vi "VI Server_Set Control Signaling Value from String Format.vi"(4 "milliseconds to wait (10 ms)":u32=10, 6 "New Signaling Value (String)":string, 7 "Label":string, 8 "error in (no error)":errorcluster, 11 "VI Server Cluster":T1={"Labels"=["Label", "Size", "Font", "Heght", "Width", "Ledding Denominator", "Ledding Nominator", "Label Number", "Microstep Resolution", "X", "Y", "Z", "Italic?", "Underlined?"], "Refs"=[], "VI Ref"=refnum}) -> (0 "error out":errorcluster, 3 "VI Server Cluster.DUP":T1={"Labels"=["Label", "Size", "Font", "Heght", "Width", "Ledding Denominator", "Ledding Nominator", "Label Number", "Microstep Resolution", "X", "Y", "Z", "Italic?", "Underlined?"], "Refs"=[], "VI Ref"=refnum})   [LabVIEW 2020, in "VI Server Toolkit LV2013.lvlib"]
doc: "<B>Set Control Values From String Formats.vi</B> and converts string values of the selected GUI objects onto original data type.\nInserts value change event into Windows Events Queue."
uses:
  VI Server Toolkit LV2013.lvlib
  VI Server_TypeDefs/VI Server_RefsCluster.ctl
panel:
  in  "Path":refnum<vi>
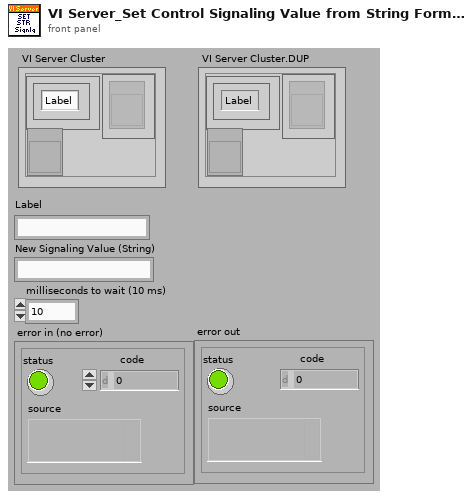
[diagram p1: front panel]
types:
  T1 = typedef "VI Server_RefsCluster.ctl" = cluster{"Labels":string[], "Refs":refnum<vi>[], "VI Ref":refnum<vi>}
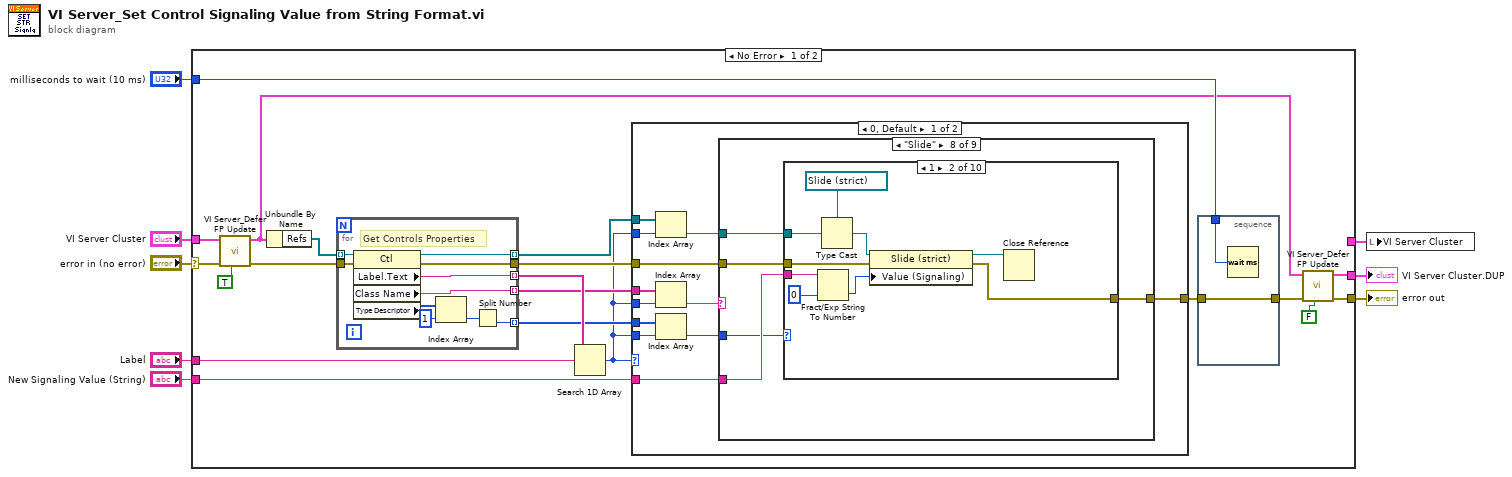
[diagram p0: block diagram]
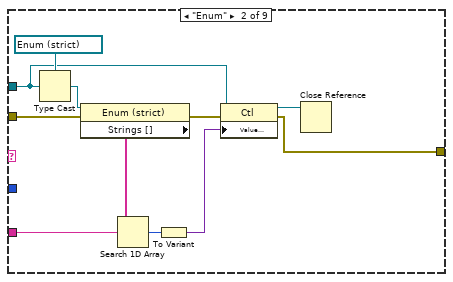
[diagram p3: hidden frame]
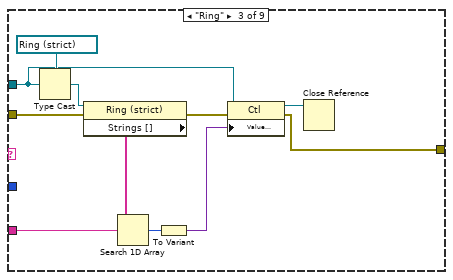
[diagram p4: hidden frame]
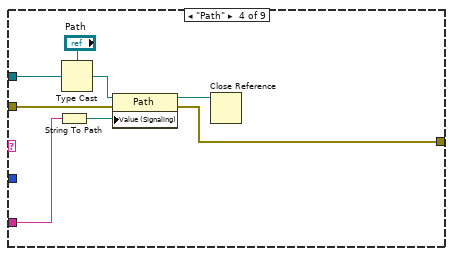
[diagram p5: hidden frame]
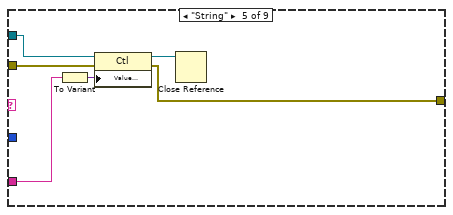
[diagram p6: hidden frame]
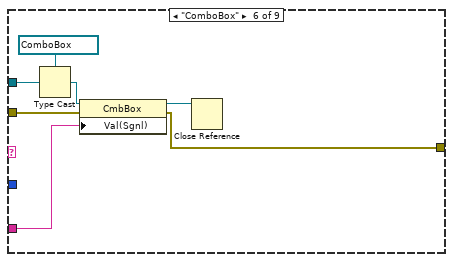
[diagram p7: hidden frame]
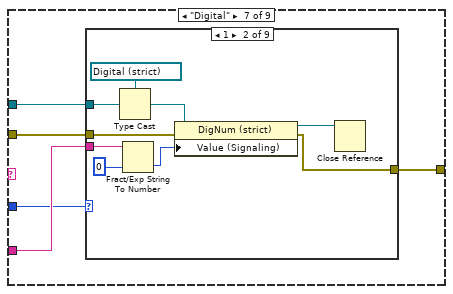
[diagram p8: hidden frame]
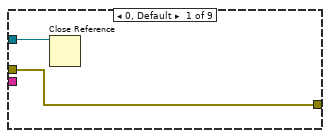
[diagram p9: hidden frame]
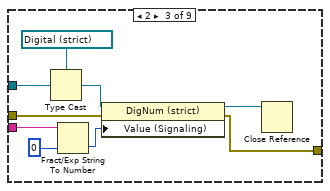
[diagram p10: hidden frame]
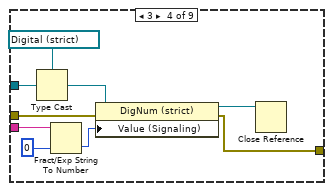
[diagram p11: hidden frame]
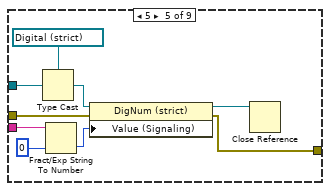
[diagram p12: hidden frame]
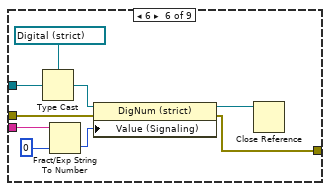
[diagram p13: hidden frame]
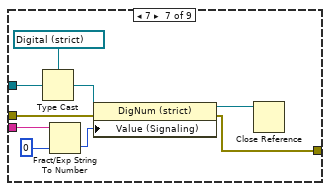
[diagram p14: hidden frame]
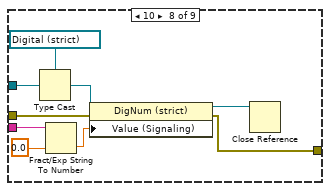
[diagram p15: hidden frame]
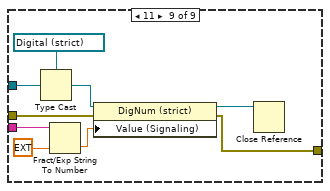
[diagram p16: hidden frame]
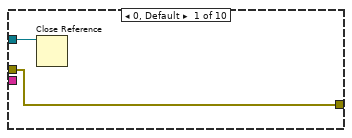
[diagram p17: hidden frame]
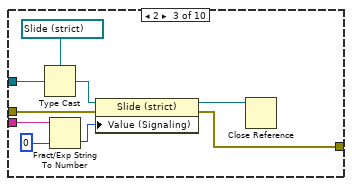
[diagram p18: hidden frame]
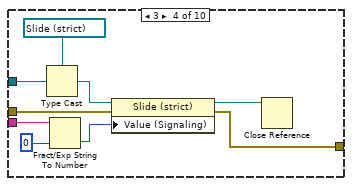
[diagram p19: hidden frame]
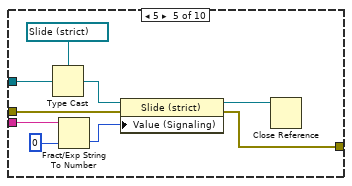
[diagram p20: hidden frame]
diagram:
  n1 = case shown="No Error" "error in (no error)" {
    selector: "error in (no error)" -> [w21 w275]
    tunnel: "New Signaling Value (String)" -> [w23 _]
    tunnel: [w17 w275] -> w8
    tunnel: "VI Server Cluster" -> [w19 _]
    tunnel: "milliseconds to wait (10 ms)" -> [w14 _]
    tunnel: "Label" -> [w13 _]
    tunnel: [w9 _] -> w2
    tunnel: [_ w274] -> w1
    frame No Error {
      n2 = call "VI Server_Defer FP Update.vi"("Defer Panel Updates? (F)"=TRUE ("Defer Panel Updates (F)"), "error in"=w21, "VI Server Cluster"=w19) -> ("error out"=w20:errorcluster, "VI Server Cluster.DUP"=w10:T1)  [unwired: 7 out]
      n3 = Unbundle By Name(w10) -> ("Refs"=w22:refnum<vi>[])
      n4 = for {
        tunnel: w22 -> [w273] mode=indexing
        tunnel: w20 -> [w272]
        tunnel: [w271] -> w28 mode=indexing
        tunnel: [w270] -> w26 mode=indexing
        tunnel: [w269] -> w27 mode=indexing
        tunnel: [w268] -> w25
        tunnel: [w264] -> w24 mode=indexing
        # "Get Controls Properties"
        n5 = property class="Ctl"(reference=w273, error in=w272) -> (reference out=w269:refnum<vi>, error out=w268:errorcluster, "Label.Text"=w271:string, "Class Name"=w270:string, "Type Descriptor"=w267:i16[])
        n6 = Index Array(array=w267, index=1) -> (element=w265:i16)
        n7 = Split Number(x=w265) -> (lo(x)=w264:u8)  [unwired: 1 out]
      }
      n8 = Search 1D Array(1D array=w28, element=w13) -> (index of element=w12:i32)  [unwired: 1 out]
      n9 = case shown="0, Default" w12 {
        tunnel: w27 -> [w42 _]
        tunnel: w12 -> [w41 _]
        tunnel: w26 -> [w40 _]
        tunnel: w12 -> [w39 _]
        tunnel: w23 -> [w36 _]
        tunnel: w25 -> [w35 w263]
        tunnel: [w34 w263] -> w11
        tunnel: w24 -> [w33 _]
        tunnel: w12 -> [w32 _]
        frame 0, Default {
          n10 = Index Array(array=w42, index=w41) -> (element=w37:refnum<vi>)
          n11 = Index Array(array=w40, index=w39) -> (element=w38:string)
          n12 = Index Array(array=w33, index=w32) -> (element=w31:u8)
          n13 = case shown="\"Slide\"" w38 {
            tunnel: w37 -> [_ w46 w55 w68 w79 w86 w89 w168 w260]
            tunnel: w36 -> [_ w52 w64 w72 w78 w80 w88 w167 w258]
            tunnel: w35 -> [w43 w49 w58 w69 w76 w84 w91 w170 w262]
            tunnel: [w43 w47 w56 w70 w75 w83 w90 w169 w261] -> w34
            tunnel: w31 -> [_ _ _ _ _ _ w87 w166 _]
            frame "", Default {
            }
            frame "Enum" {
              n14 = Type Cast(type=refnum<vi> refnum ("Enum"), x=w46) -> (*(type *) &x=w53:refnum<vi>)
              n15 = property class="Enum (strict)"(reference=w53, error in=w49) -> (error out=w48:errorcluster, "Strings []"=w51:string[])  [unwired: 1 out]
              n16 = Search 1D Array(1D array=w51, element=w52) -> (index of element=w45:i32)  [unwired: 1 out]
              n17 = To Variant(anything=w45) -> (Variant=w44:variant)
              n18 = property class="Ctl"(reference=w46, error in=w48, "Value (Signaling)"=w44) -> (reference out=w50:refnum<vi>, error out=w47:errorcluster)
              n19 = Close Reference(reference=w50) -> ()  [unwired: 1 in, 1 out]
            }
            frame "Ring" {
              n20 = Type Cast(type=refnum<vi> refnum ("Ring"), x=w55) -> (*(type *) &x=w65:refnum<vi>)
              n21 = property class="Ring (strict)"(reference=w65, error in=w58) -> (error out=w57:errorcluster, "Strings []"=w62:string[])  [unwired: 1 out]
              n22 = Search 1D Array(1D array=w62, element=w64) -> (index of element=w63:i32)  [unwired: 1 out]
              n23 = To Variant(anything=w63) -> (Variant=w61:variant)
              n24 = property class="Ctl"(reference=w55, error in=w57, "Value (Signaling)"=w61) -> (reference out=w60:refnum<vi>, error out=w56:errorcluster)
              n25 = Close Reference(reference=w60) -> ()  [unwired: 1 in, 1 out]
            }
            frame "Path" {
              n26 = String To Path(string=w72) -> (path=w73:path)
              n27 = Type Cast(type="Path", x=w68) -> (*(type *) &x=w67:refnum<vi>)
              n28 = property class="Path"(reference=w67, error in=w69, "Value (Signaling)"=w73) -> (reference out=w71:refnum<vi>, error out=w70:errorcluster)
              n29 = Close Reference(reference=w71) -> ()  [unwired: 1 in, 1 out]
            }
            frame "String" {
              n30 = To Variant(anything=w78) -> (Variant=w74:variant)
              n31 = property class="Ctl"(reference=w79, error in=w76, "Value (Signaling)"=w74) -> (reference out=w77:refnum<vi>, error out=w75:errorcluster)
              n32 = Close Reference(reference=w77) -> ()  [unwired: 1 in, 1 out]
            }
            frame "ComboBox" {
              n33 = Type Cast(type=refnum<vi> refnum ("TDS.TriggerType"), x=w86) -> (*(type *) &x=w82:refnum<vi>)
              n34 = property class="CmbBox"(reference=w82, error in=w84, "Val(Sgnl)"=w80) -> (reference out=w85:refnum<vi>, error out=w83:errorcluster)
              n35 = Close Reference(reference=w85) -> ()  [unwired: 1 in, 1 out]
            }
            frame "Digital" {
              n36 = case shown="1" w87 {
                tunnel: w91 -> [w93 w102 w109 w115 w125 w133 w144 w151 w162]
                tunnel: [w93 w101 w106 w117 w127 w135 w142 w153 w161] -> w90
                tunnel: w89 -> [w92 w100 w111 w120 w129 w138 w147 w156 w165]
                tunnel: w88 -> [_ w98 w108 w116 w124 w134 w143 w152 w160]
                frame 0, Default {
                  n37 = Close Reference(reference=w92) -> ()  [unwired: 1 in, 1 out]
                }
                frame 1 {
                  n38 = Type Cast(type=refnum<vi> refnum ("I8"), x=w100) -> (*(type *) &x=w99:refnum<vi>)
                  n39 = Fract/Exp String To Number(string=w98, default (0 dbl)=i8 0) -> (number=w95:i8)  [unwired: 3 out]
                  n40 = property class="DigNum (strict)"(reference=w99, error in=w102, "Value (Signaling)"=w95) -> (reference out=w96:refnum<vi>, error out=w101:errorcluster)
                  n41 = Close Reference(reference=w96) -> ()  [unwired: 1 in, 1 out]
                }
                frame 2 {
                  n42 = Type Cast(type=refnum<vi> refnum ("I16"), x=w111) -> (*(type *) &x=w107:refnum<vi>)
                  n43 = Fract/Exp String To Number(string=w108, default (0 dbl)=i16 0) -> (number=w104:i16)  [unwired: 3 out]
                  n44 = property class="DigNum (strict)"(reference=w107, error in=w109, "Value (Signaling)"=w104) -> (reference out=w105:refnum<vi>, error out=w106:errorcluster)
                  n45 = Close Reference(reference=w105) -> ()  [unwired: 1 in, 1 out]
                }
                frame 3 {
                  n46 = Type Cast(type=refnum<vi> refnum ("I32"), x=w120) -> (*(type *) &x=w118:refnum<vi>)
                  n47 = Fract/Exp String To Number(string=w116, default (0 dbl)=0) -> (number=w113:i32)  [unwired: 3 out]
                  n48 = property class="DigNum (strict)"(reference=w118, error in=w115, "Value (Signaling)"=w113) -> (reference out=w114:refnum<vi>, error out=w117:errorcluster)
                  n49 = Close Reference(reference=w114) -> ()  [unwired: 1 in, 1 out]
                }
                frame 5 {
                  n50 = Type Cast(type=refnum<vi> refnum ("U8"), x=w129) -> (*(type *) &x=w126:refnum<vi>)
                  n51 = Fract/Exp String To Number(string=w124, default (0 dbl)=u8 0) -> (number=w122:u8)  [unwired: 3 out]
                  n52 = property class="DigNum (strict)"(reference=w126, error in=w125, "Value (Signaling)"=w122) -> (reference out=w123:refnum<vi>, error out=w127:errorcluster)
                  n53 = Close Reference(reference=w123) -> ()  [unwired: 1 in, 1 out]
                }
                frame 6 {
                  n54 = Type Cast(type=refnum<vi> refnum ("U16"), x=w138) -> (*(type *) &x=w136:refnum<vi>)
                  n55 = Fract/Exp String To Number(string=w134, default (0 dbl)=u16 0) -> (number=w131:u16)  [unwired: 3 out]
                  n56 = property class="DigNum (strict)"(reference=w136, error in=w133, "Value (Signaling)"=w131) -> (reference out=w132:refnum<vi>, error out=w135:errorcluster)
                  n57 = Close Reference(reference=w132) -> ()  [unwired: 1 in, 1 out]
                }
                frame 7 {
                  n58 = Type Cast(type=refnum<vi> refnum ("U32"), x=w147) -> (*(type *) &x=w145:refnum<vi>)
                  n59 = Fract/Exp String To Number(string=w143, default (0 dbl)=u32 0) -> (number=w140:u32)  [unwired: 3 out]
                  n60 = property class="DigNum (strict)"(reference=w145, error in=w144, "Value (Signaling)"=w140) -> (reference out=w141:refnum<vi>, error out=w142:errorcluster)
                  n61 = Close Reference(reference=w141) -> ()  [unwired: 1 in, 1 out]
                }
                frame 10 {
                  n62 = Type Cast(type=refnum<vi> refnum ("DBL"), x=w156) -> (*(type *) &x=w154:refnum<vi>)
                  n63 = Fract/Exp String To Number(string=w152, default (0 dbl)=0.0) -> (number=w149:dbl)  [unwired: 3 out]
                  n64 = property class="DigNum (strict)"(reference=w154, error in=w151, "Value (Signaling)"=w149) -> (reference out=w150:refnum<vi>, error out=w153:errorcluster)
                  n65 = Close Reference(reference=w150) -> ()  [unwired: 1 in, 1 out]
                }
                frame 11 {
                  n66 = Type Cast(type=refnum<vi> refnum ("EXT"), x=w165) -> (*(type *) &x=w163:refnum<vi>)
                  n67 = Fract/Exp String To Number(string=w160, default (0 dbl)=ext 0.0) -> (number=w158:ext)  [unwired: 3 out]
                  n68 = property class="DigNum (strict)"(reference=w163, error in=w162, "Value (Signaling)"=w158) -> (reference out=w159:refnum<vi>, error out=w161:errorcluster)
                  n69 = Close Reference(reference=w159) -> ()  [unwired: 1 in, 1 out]
                }
              }
            }
            frame "Slide" {
              n70 = case shown="1" w166 {
                tunnel: w170 -> [w172 w178 w188 w195 w205 w213 w223 w232 w241 w250]
                tunnel: [w172 w179 w189 w197 w203 w214 w221 w230 w239 w248] -> w169
                tunnel: w168 -> [w171 w181 w190 w199 w208 w217 w226 w235 w244 w253]
                tunnel: w167 -> [_ w177 w186 w194 w204 w212 w222 w231 w240 w249]
                frame 0, Default {
                  n71 = Close Reference(reference=w171) -> ()  [unwired: 1 in, 1 out]
                }
                frame 1 {
                  n72 = Fract/Exp String To Number(string=w177, default (0 dbl)=u8 0) -> (number=w173:u8)  [unwired: 3 out]
                  n73 = Type Cast(type=refnum<vi> refnum ("Slide"), x=w181) -> (*(type *) &x=w180:refnum<vi>)
                  n74 = property class="Slide (strict)"(reference=w180, error in=w178, "Value (Signaling)"=w173) -> (reference out=w175:refnum<vi>, error out=w179:errorcluster)
                  n75 = Close Reference(reference=w175) -> ()  [unwired: 1 in, 1 out]
                }
                frame 2 {
                  n76 = Type Cast(type=refnum<vi> refnum ("Slide"), x=w190) -> (*(type *) &x=w187:refnum<vi>)
                  n77 = Fract/Exp String To Number(string=w186, default (0 dbl)=u16 0) -> (number=w183:u16)  [unwired: 3 out]
                  n78 = property class="Slide (strict)"(reference=w187, error in=w188, "Value (Signaling)"=w183) -> (reference out=w184:refnum<vi>, error out=w189:errorcluster)
                  n79 = Close Reference(reference=w184) -> ()  [unwired: 1 in, 1 out]
                }
                frame 3 {
                  n80 = Type Cast(type=refnum<vi> refnum ("Slide"), x=w199) -> (*(type *) &x=w196:refnum<vi>)
                  n81 = Fract/Exp String To Number(string=w194, default (0 dbl)=0) -> (number=w192:i32)  [unwired: 3 out]
                  n82 = property class="Slide (strict)"(reference=w196, error in=w195, "Value (Signaling)"=w192) -> (reference out=w193:refnum<vi>, error out=w197:errorcluster)
                  n83 = Close Reference(reference=w193) -> ()  [unwired: 1 in, 1 out]
                }
                frame 5 {
                  n84 = Type Cast(type=refnum<vi> refnum ("Slide"), x=w208) -> (*(type *) &x=w206:refnum<vi>)
                  n85 = Fract/Exp String To Number(string=w204, default (0 dbl)=u8 0) -> (number=w201:u8)  [unwired: 3 out]
                  n86 = property class="Slide (strict)"(reference=w206, error in=w205, "Value (Signaling)"=w201) -> (reference out=w202:refnum<vi>, error out=w203:errorcluster)
                  n87 = Close Reference(reference=w202) -> ()  [unwired: 1 in, 1 out]
                }
                frame 6 {
                  n88 = Fract/Exp String To Number(string=w212, default (0 dbl)=u16 0) -> (number=w210:u16)  [unwired: 3 out]
                  n89 = Type Cast(type=refnum<vi> refnum ("Slide"), x=w217) -> (*(type *) &x=w215:refnum<vi>)
                  n90 = property class="Slide (strict)"(reference=w215, error in=w213, "Value (Signaling)"=w210) -> (reference out=w211:refnum<vi>, error out=w214:errorcluster)
                  n91 = Close Reference(reference=w211) -> ()  [unwired: 1 in, 1 out]
                }
                frame 7 {
                  n92 = Type Cast(type=refnum<vi> refnum ("Slide"), x=w226) -> (*(type *) &x=w224:refnum<vi>)
                  n93 = Fract/Exp String To Number(string=w222, default (0 dbl)=u32 0) -> (number=w219:u32)  [unwired: 3 out]
                  n94 = property class="Slide (strict)"(reference=w224, error in=w223, "Value (Signaling)"=w219) -> (reference out=w220:refnum<vi>, error out=w221:errorcluster)
                  n95 = Close Reference(reference=w220) -> ()  [unwired: 1 in, 1 out]
                }
                frame 9 {
                  n96 = Fract/Exp String To Number(string=w231, default (0 dbl)=sgl 0.0) -> (number=w228:sgl)  [unwired: 3 out]
                  n97 = Type Cast(type=refnum<vi> refnum ("Slide"), x=w235) -> (*(type *) &x=w233:refnum<vi>)
                  n98 = property class="Slide (strict)"(reference=w233, error in=w232, "Value (Signaling)"=w228) -> (reference out=w229:refnum<vi>, error out=w230:errorcluster)
                  n99 = Close Reference(reference=w229) -> ()  [unwired: 1 in, 1 out]
                }
                frame 10 {
                  n100 = Fract/Exp String To Number(string=w240, default (0 dbl)=0.0) -> (number=w237:dbl)  [unwired: 3 out]
                  n101 = Type Cast(type=refnum<vi> refnum ("Slide"), x=w244) -> (*(type *) &x=w242:refnum<vi>)
                  n102 = property class="Slide (strict)"(reference=w242, error in=w241, "Value (Signaling)"=w237) -> (reference out=w238:refnum<vi>, error out=w239:errorcluster)
                  n103 = Close Reference(reference=w238) -> ()  [unwired: 1 in, 1 out]
                }
                frame 11 {
                  n104 = Fract/Exp String To Number(string=w249, default (0 dbl)=ext 0.0) -> (number=w246:ext)  [unwired: 3 out]
                  n105 = Type Cast(type=refnum<vi> refnum ("Slide"), x=w253) -> (*(type *) &x=w251:refnum<vi>)
                  n106 = property class="Slide (strict)"(reference=w251, error in=w250, "Value (Signaling)"=w246) -> (reference out=w247:refnum<vi>, error out=w248:errorcluster)
                  n107 = Close Reference(reference=w247) -> ()  [unwired: 1 in, 1 out]
                }
              }
            }
            frame "Boolean" {
              n108 = Type Cast(type=refnum<vi> refnum ("Boolean 2"), x=w260) -> (*(type *) &x=w259:refnum<vi>)
              n109 = Equal?(x=w258, y="TRUE" ("x")) -> (x = y?=w255:bool)
              n110 = property class="Bool (strict)"(reference=w259, error in=w262, "Value (Signaling)"=w255) -> (reference out=w256:refnum<vi>, error out=w261:errorcluster)
              n111 = Close Reference(reference=w256) -> ()  [unwired: 1 in, 1 out]
            }
          }
        }
        frame -1 {
        }
      }
      n112 = stacked-sequence {
        tunnel: w11 -> [w30]
        tunnel: [w30] -> w16
        tunnel: w14 -> [w29]
        frame #0 {
          n113 = Wait (ms)(milliseconds to wait=w29) -> ()  [unwired: 1 out]
        }
      }
      n114 = call "VI Server_Defer FP Update.vi"("Defer Panel Updates? (F)"=FALSE ("Defer Panel Updates (F)"), "error in"=w16, "VI Server Cluster"=w10) -> ("error out"=w17:errorcluster, "VI Server Cluster.DUP"=w9:T1)  [unwired: 7 out]
    }
    frame Error {
      n115 = call "VI Server_Empty VI Server Cluster.vi"() -> ("VI Server Cluster"=w274:T1)  [unwired: 7 in]
    }
  }
  "error out" <- w8
  "VI Server Cluster.DUP" <- w2
  n116 = local write "VI Server Cluster"(w1) -> ()
